vi "Draw Image to Picture (ARGB).vi"(7 "Image Draw Offset (Default 0,0)":T1, 8 "error in (no error)":errorcluster, 11 "ARGB Image Source in":T2) -> (0 "error out":errorcluster, 3 "Picture":picture)   [LabVIEW 2020, in "image.lvlib"]
doc: "Draw an image to a LabVIEW Picture."
uses:
  image.lvlib
  ARGB Image.ctl
  Image Draw Offset.ctl
  8cd07b1b-062e-4fe4-9e87-2eb3dc89fe0e.vi
  <vilib>/Utility/error.llb/Error Cluster From Error Code.vi
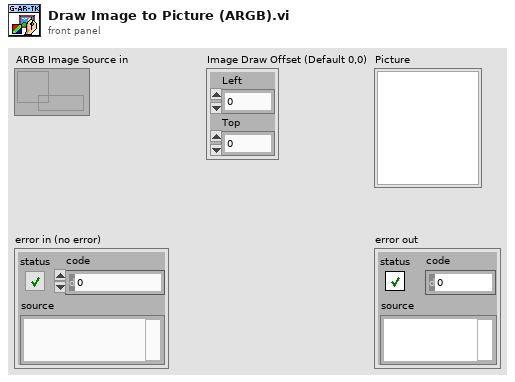
[diagram p1: front panel]
types:
  T1 = typedef "image.lvlib/Image Draw Offset.ctl" = cluster{"Left":i16, "Top":i16}
  T2 = typedef "image.lvlib/ARGB Image.ctl" = refnum<data-value>
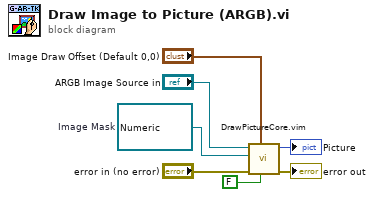
[diagram p0: block diagram]
diagram:
  w1 = refnum<data-value> refnum  # Image Mask
  n1 = call "DrawPictureCore.vim"("HasMask"=FALSE, "Image Draw Offset"="Image Draw Offset (Default 0,0)", "error in (no error)"="error in (no error)", "Image Mask"=w1, "Image Src"="ARGB Image Source in") -> ("error out"=→"error out":errorcluster, "Picture"=→"Picture":picture)  [unwired: 5 in]
